vi "UpdateOneError.vi"(4 "Description":string, 6 "Library":string, 8 "ErrorIn":errorcluster caption="Error In(no Error)", 9 "Text":string, 10 "ErrorCode":i32, 11 "ReferenceIn":refnum<class "ErrorDefinitionSQLite.lvclass"> caption="Reference In") -> (0 "ErrorOut":errorcluster caption="Error Out", 3 "ReferenceOut":refnum<class "ErrorDefinitionSQLite.lvclass"> caption="Reference Out")   [LabVIEW 2018, in "ErrorDefinitionSQLite.lvclass"]
uses:
  <userlib>/_express/CustomErrorCreator/ErrorDefinitionSQLite/ErrorDefinitionSQLite.lvclass
  <vilib>/drjdpowell/SQLite Library/SQL Connection/Open (path).vi
  <vilib>/drjdpowell/SQLite Library/SQL Connection/Open (string).vi
  <vilib>/AdvancedString/Path To Command Line String.vi
  <vilib>/drjdpowell/SQLite Library/SQL Connection/Execute SQL.vi
  <vilib>/drjdpowell/SQLite Library/SQL Connection/Connection.lvclass
  <vilib>/drjdpowell/SQLite Library/SQLite.lvlib
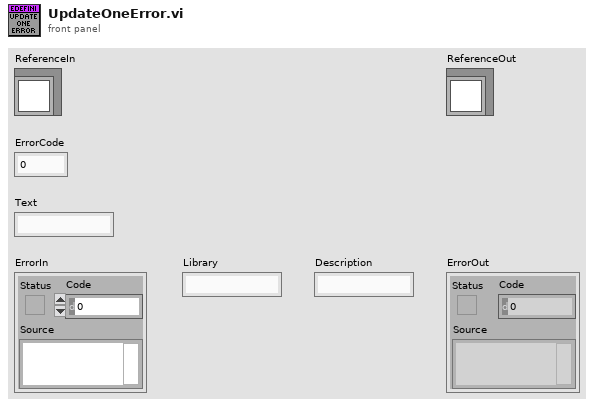
[diagram p1: front panel]
types:
  T1 = enum16{"New or existing", "Existing", "Read only"}
  T2 = typedef "ErrorDefinitionSQLite.lvclass/ObjectAttributes.ctl" = cluster{"Path":path}
  T3 = cluster{"Text":string, "Library":string, "Description":string, "App.UserName":string}
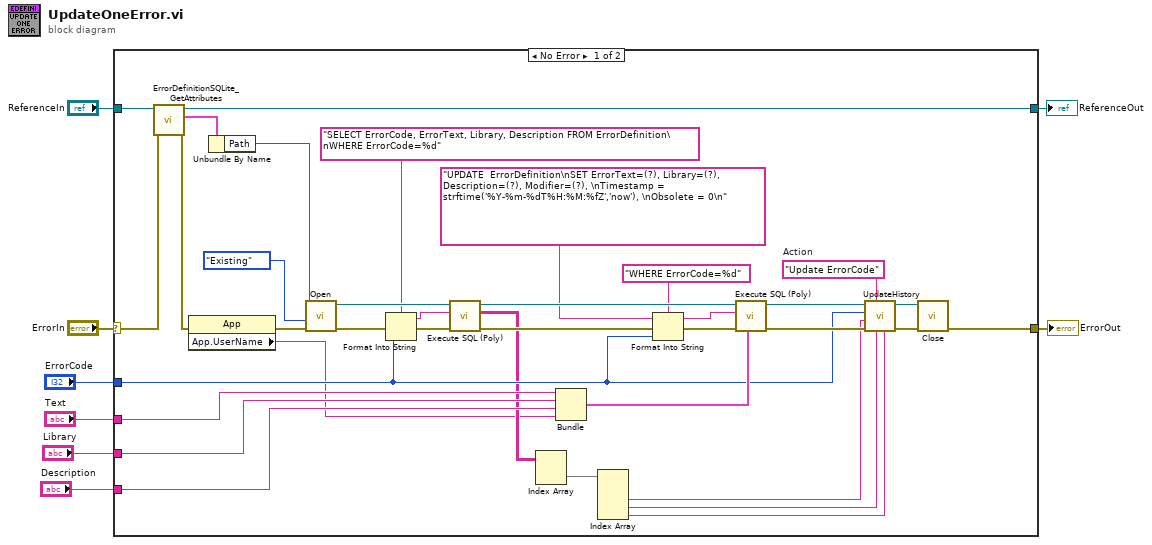
[diagram p0: block diagram]
diagram:
  n1 = case shown="No Error" "ErrorIn" {
    selector: "ErrorIn" -> [w44 w46]
    tunnel: [w38 w46] -> w7
    tunnel: [w42 w45] -> w5
    tunnel: "ReferenceIn" -> [w43 w45]
    tunnel: "ErrorCode" -> [w20 _]
    tunnel: "Text" -> [w29 _]
    tunnel: "Library" -> [w28 _]
    tunnel: "Description" -> [w27 _]
    frame No Error {
      w34 = "Update ErrorCode"  # Action
      n2 = call <userlib>:"ErrorDefinitionSQLite_GetAttributes.vi"("ErrorIn"=w44, "Reference in"=w43) -> ("ErrorOut"=w13:errorcluster, "Data"=w40:T2, "Reference out"=w42:refnum<class "ErrorDefinitionSQLite.lvclass">)  [unwired: 6 in, 1 out]
      n3 = property class="App"(error in=w13) -> (error out=w12:errorcluster, "App.UserName"=w9:string)  [unwired: 1 in, 1 out]
      n4 = Unbundle By Name(w40) -> ("Path"=w39:path)
      n5 = call-poly <vilib>:"Open.vi"("error in (no error)"=w12, "File Option"=T1."Existing", "db file"=w39) -> ("error out"=w22:errorcluster, "SQLite Connection"=w26:refnum<class "Connection.lvclass">)  [unwired: 7 in]
      n6 = Format Into String(format string="SELECT ErrorCode, ErrorText, Library, Description FROM ErrorDefinition\nWHERE ErrorCode=%d" ("SQL"), error in=w22, w20) -> (resulting string=w19:string, error out=w21:errorcluster)  [unwired: 1 in]
      n7 = call-poly <vilib>:"Execute SQL (Poly).vi"("error in (no error)"=w21, "SQL"=w19, "SQLite Connection in"=w26) -> ("error out"=w25:errorcluster, "Result Set"=w18:string[][], "SQLite Connection"=w24:refnum<class "Connection.lvclass">)  [unwired: 5 in, 1 out]
      n8 = Index Array(array=w18) -> (element=w17:string[])  [unwired: 2 in]
      n9 = Bundle("Text"=w29, "Library"=w28, "Description"=w27, "App.UserName"=w9) -> (w35:T3)  [unwired: 1 in]
      n10 = Index Array(array=w17) -> (element #2=w16:string, element #3=w15:string, element #4=w14:string)  [unwired: 4 in, 1 out]
      n11 = Format Into String(format string="WHERE ErrorCode=%d" ("SQL"), initial string="UPDATE  ErrorDefinition\nSET ErrorText=(?), Library=(?), Description=(?), Modifier=(?), \nTimestamp = strftime('%Y-%m-%dT%H:%M:%fZ','now'), \nObsolete = 0\n" ("SQL"), error in=w25, w20) -> (resulting string=w36:string, error out=w37:errorcluster)
      n12 = call-poly <vilib>:"Execute SQL (Poly).vi"("Parameter(s)"=w35, "error in (no error)"=w37, "SQL"=w36, "SQLite Connection in"=w24) -> ("error out"=w30:errorcluster, "SQLite Connection"=w33:refnum<class "Connection.lvclass">)  [unwired: 4 in, 2 out]
      n13 = call <userlib>:"UpdateHistory.vi"("Description"=w14, "Library"=w15, "Action"=w34, "error in (no error)"=w30, "ErrorText"=w16, "ErrorCode"=w20, "Connection in"=w33) -> ("error out"=w31:errorcluster, "Connection out"=w32:refnum<class "Connection.lvclass">)  [unwired: 3 in]
      n14 = call-dynamic "Close.vi"("error in (no error)"=w31, "SQLite Connection in"=w32) -> ("error out"=w38:errorcluster)  [unwired: 9 in]
    }
    frame Error {
    }
  }
  "ErrorOut" <- w7
  "ReferenceOut" <- w5
